vi "TCPRead_Write.vi"(9 "String":string, 10 "error out 2":errorcluster, 11 "connection ID 2":refnum<k5>) -> (2 "error out":errorcluster, 3 "connection ID":refnum<k5>)   [LabVIEW 2016]
uses:
  TCPRead_Write_GlobalVariables.vi
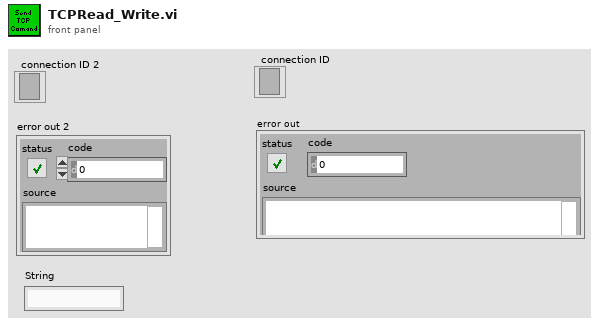
[diagram p1: front panel]
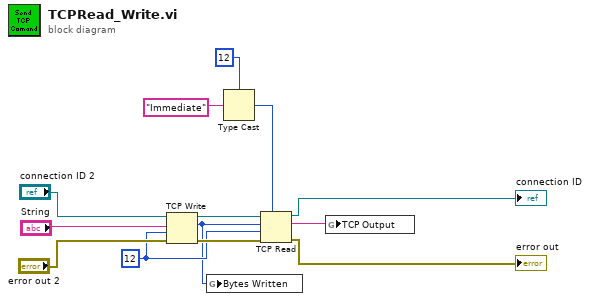
[diagram p0: block diagram]
diagram:
  w5 = 12
  n1 = TCP Write(connection ID="connection ID 2", data in="String", error in (no error)="error out 2", 9:w5) -> (connection ID out=w13:refnum<k5>, bytes written=w1:i32, error out=w12:errorcluster)
  n2 = global write "TCPRead_Write_GlobalVariables.vi" "Bytes Written"(w1) -> ()
  n3 = Type Cast(type=u16 12, x="Immediate") -> (*(type *) &x=w3:u16)
  n4 = TCP Read(connection ID=w13, bytes to read=w1, error in (no error)=w12, 7:w3, 9:w5) -> (connection ID out=→"connection ID":refnum<k5>, data out=w7:string, error out=→"error out":errorcluster)
  n5 = global write "TCPRead_Write_GlobalVariables.vi" "TCP Output"(w7) -> ()
